vi "最小试剂余量百分比.vi"   [LabVIEW 2016, in "斯坦道CODMn新电路板.lvlib"]
uses:
  <vilib>/Analysis/BLAS.llb/izamin - Min Element Index (CDB).vi
  <vilib>/Analysis/NI_AALBLAS.lvlib
types:
  T1 = cluster{"V1":sgl, "V2":sgl, "V3":sgl, "V4":sgl, "V5":sgl, "V6":sgl, "V7":sgl, "V8":sgl, "V9":sgl, "V10":sgl, "V11":sgl, "V12":sgl, "V9-1":sgl, "V9-2":sgl}
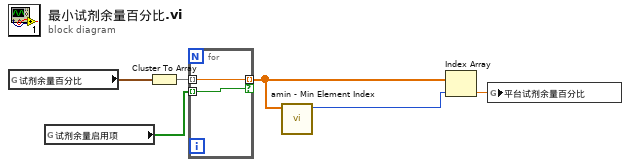
[diagram p0: block diagram]
diagram:
  n1 = global read "VARCODMn全局变量.vi" "试剂余量百分比"() -> (w3:T1)
  n2 = global read "VARCODMn全局变量.vi" "试剂余量启用项"() -> (w2:bool[])
  n3 = Cluster To Array(cluster=w3) -> (array=w5:sgl[])
  n4 = for {
    tunnel: w5 -> [w8] mode=indexing
    tunnel: w2 -> [w7] mode=indexing
    tunnel: [w8] -> w4 mode=indexing if=w7
  }
  n5 = call-poly <vilib>:"amin - Min Element Index.vi"("x"=w4) -> ("izamin"=w6:i32)  [unwired: 9 in, 1 out]
  n6 = Index Array(array=w4, index=w6) -> (element=w1:sgl)
  n7 = global write "VARCODMn全局变量.vi" "平台试剂余量百分比"(w1) -> ()
